vi "window_graph  feature_value2string.vi"(1 "feature cluster":T1) -> (0 "feature string":string)   [LabVIEW 2018]
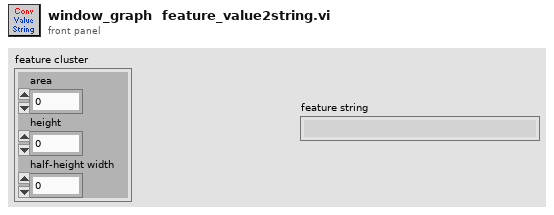
[diagram p1: front panel]
types:
  T1 = cluster{"area":dbl, "height":dbl, "half-height width":dbl}
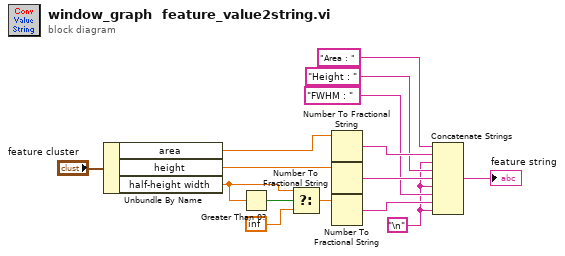
[diagram p0: block diagram]
diagram:
  w7 = "\n"
  n1 = Unbundle By Name("feature cluster") -> ("area"=w15:dbl, "height"=w14:dbl, "half-height width"=w2:dbl)
  n2 = Greater Than 0?(x=w2) -> (x > 0?=w5:bool)
  n3 = Select(t=w2, s=w5, f=inf) -> (s? t:f=w3:dbl)
  n4 = Number To Fractional String(number=w15) -> (F-format string=w12:string)  [unwired: 3 in]
  n5 = Number To Fractional String(number=w14) -> (F-format string=w10:string)  [unwired: 3 in]
  n6 = Number To Fractional String(number=w3) -> (F-format string=w8:string)  [unwired: 3 in]
  n7 = Concatenate Strings("Area : ", w12, w7, "Height : ", w10, w7, "FWHM : ", w8, w7) -> (→"feature string":string)
